vi "GetControlSpecificLocalizedPhrase.vi"(7 "Dictionary":T2, 8 "error in (no error)":errorcluster, 9 "Font Info":T1, 10 "Target Language":string, 11 "Control Reference":refnum<vi>) -> (0 "error out":errorcluster, 3 "Control ref out":refnum<vi>)   [LabVIEW 2019]
uses:
  Dictionary--Cluster.ctl
  Font -- Cluster.ctl
  Phrase Dictionary Entry -- Cluster.ctl
  Font Info -- Cluster.ctl
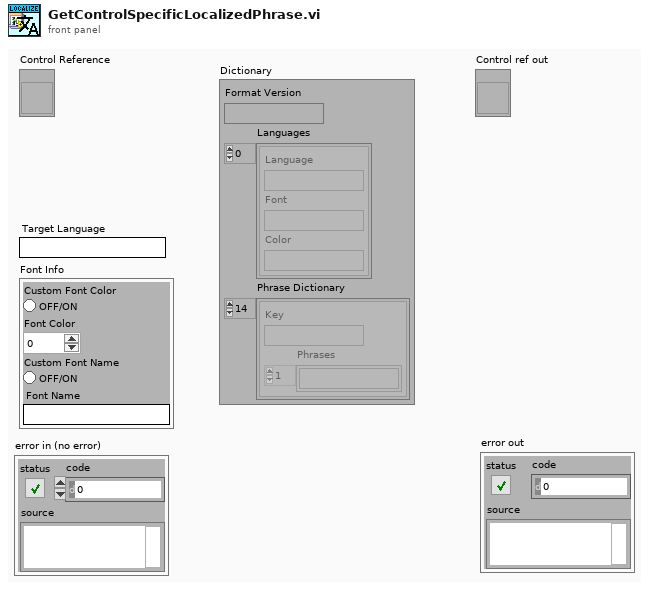
[diagram p1: front panel]
types:
  T1 = typedef "Font Info -- Cluster.ctl" = cluster{"Custom Font Color":bool, "Font Color":u32, "Custom Font Name":bool, "Font Name":string}
  T2 = typedef "Dictionary--Cluster.ctl" = cluster{"Format Version":string, "Languages":T3[], "Phrase Dictionary":T4[]}
  T3 = typedef "Font -- Cluster.ctl" = cluster{"Language":string, "Font":string, "Color":string}
  T4 = typedef "Phrase Dictionary Entry -- Cluster.ctl" = cluster{"Key":string, "Phrases":string[]}
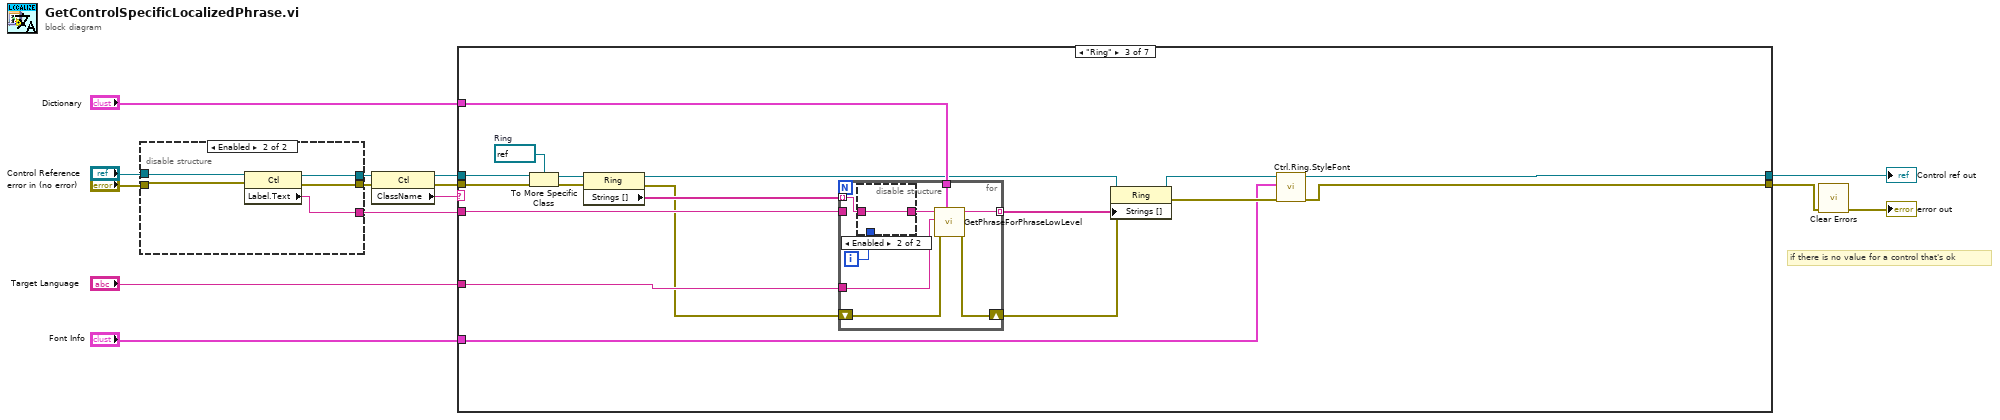
[diagram p0: block diagram]
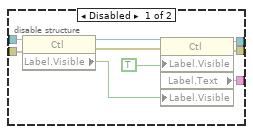
[diagram p2: hidden frame]
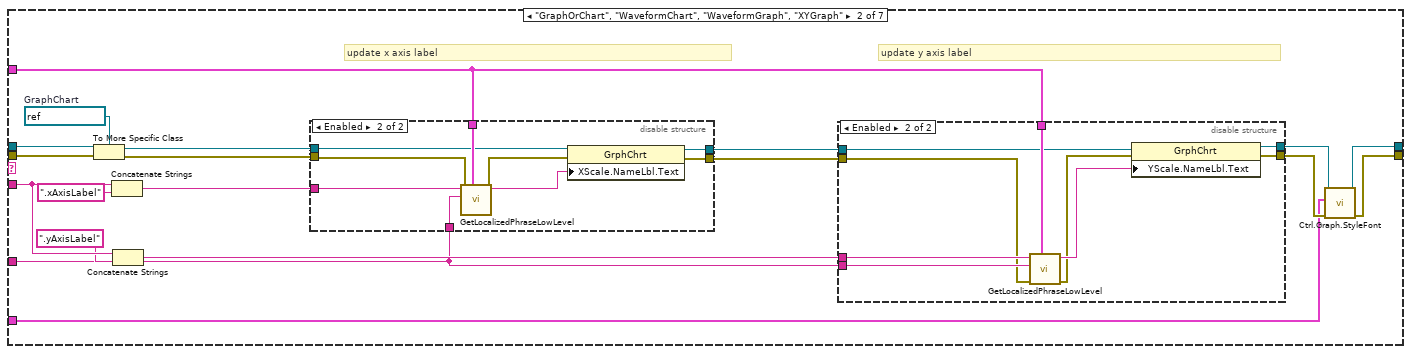
[diagram p4: hidden frame]
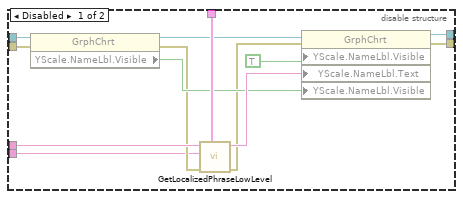
[diagram p5: hidden frame]
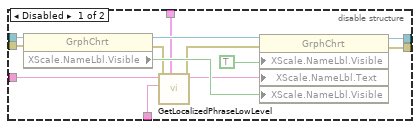
[diagram p6: hidden frame]
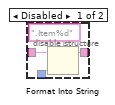
[diagram p7: hidden frame]
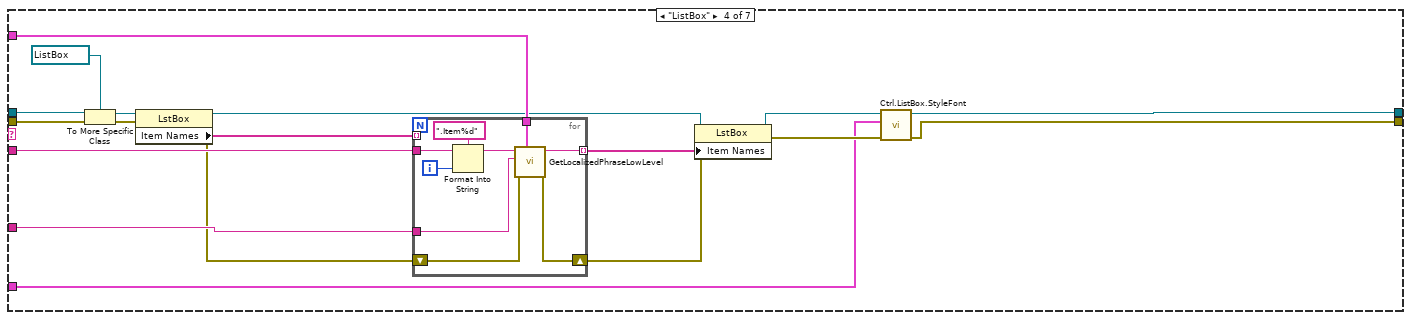
[diagram p8: hidden frame]
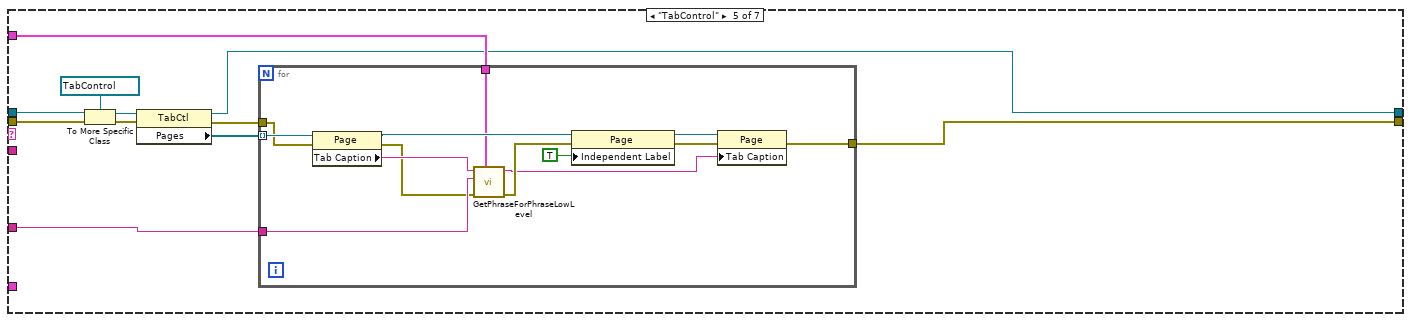
[diagram p9: hidden frame]
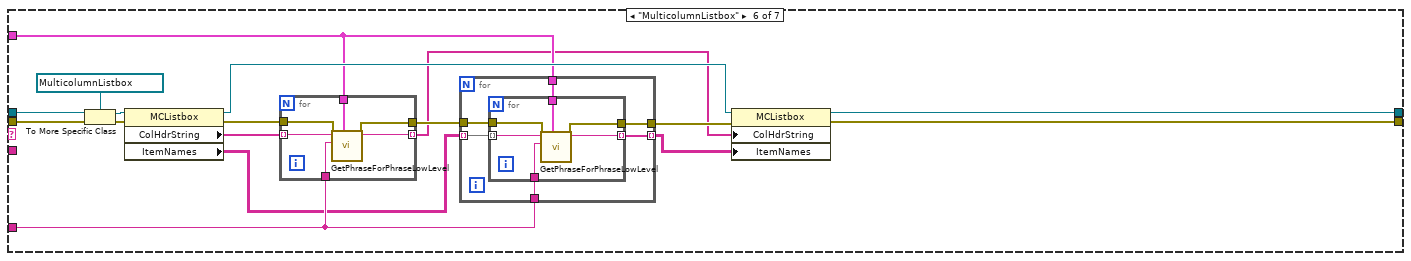
[diagram p10: hidden frame]
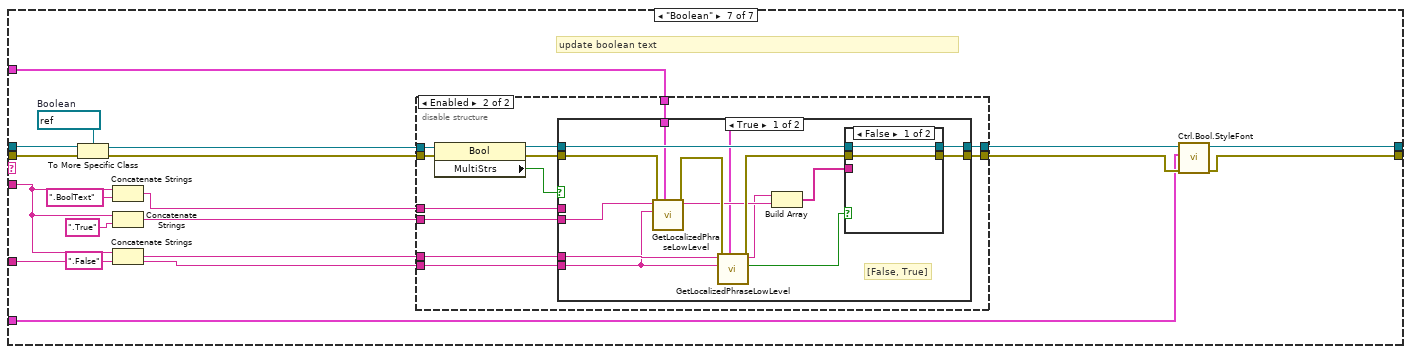
[diagram p11: hidden frame]
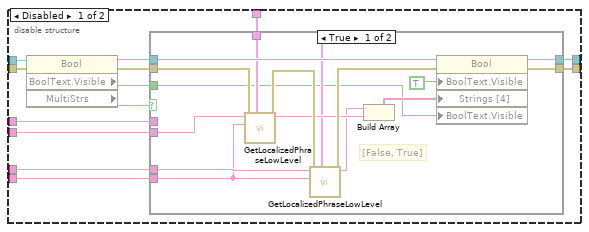
[diagram p12: hidden frame]
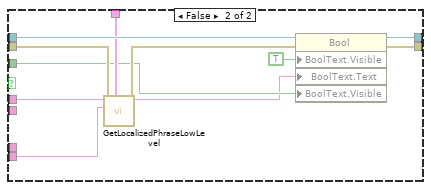
[diagram p13: hidden frame]
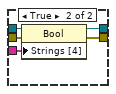
[diagram p14: hidden frame]
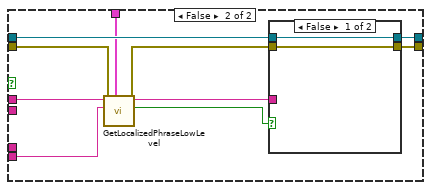
[diagram p15: hidden frame]
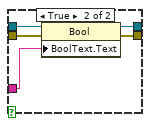
[diagram p16: hidden frame]
diagram:
  # "if there is no value for a control that's ok"
  n1 = disable-structure shown="Enabled" {
    disable-tunnel: "Control Reference" -> [w19 w24]
    disable-tunnel: [w18 w28] -> w12
    disable-tunnel: [w17 w27] -> w11
    disable-tunnel: [w16 w26] -> w8
    disable-tunnel: "error in (no error)" -> [w15 w25]
    frame Disabled {
      n2 = property on="Property Node" class="Ctl"(reference=w19, error in=w15) -> (reference out=w23:refnum<vi>, error out=w20:errorcluster, "Label.Visible"=w22:bool)
      n3 = property on="Property Node" class="Ctl"(reference=w23, error in=w20, "Label.Visible"=TRUE, "Label.Visible"=w22) -> (reference out=w18:refnum<vi>, error out=w16:errorcluster, "Label.Text"=w17:string)
    }
    frame Enabled {
      n4 = property on="Property Node" class="Ctl"(reference=w24, error in=w25) -> (reference out=w28:refnum<vi>, error out=w26:errorcluster, "Label.Text"=w27:string)
    }
  }
  n5 = property on="Property Node" class="Ctl"(reference=w12, error in=w8) -> (reference out=w10:refnum<vi>, error out=w7:errorcluster, "ClassName"=w14:string)
  n6 = case shown="\"Ring\"" w14 {
    tunnel: w11 -> [_ w44 w105 w137 _ _ w213]
    tunnel: w10 -> [w30 w48 w110 w142 w162 w192 w229]
    tunnel: "Dictionary" -> [_ w41 w104 w136 w155 w180 w222]
    tunnel: "Target Language" -> [_ w38 w103 w135 w156 w179 w221]
    tunnel: w7 -> [w29 w40 w109 w141 w161 w191 w224]
    tunnel: [w30 w35 w97 w127 w154 w185 w219] -> w6
    tunnel: [w29 w33 w95 w128 w152 w183 w217] -> w3
    tunnel: "Font Info" -> [_ w32 w94 w125 _ _ w216]
    frame "0", Default {
    }
    frame "GraphOrChart", "WaveformChart", "WaveformGraph", "XYGraph" {
      w46 = refnum<vi> refnum  # GraphChart
      # "update y axis label"
      # "update x axis label"
      n7 = To More Specific Class(target class=w46, reference=w48, error in=w40) -> (specific class reference=w47:refnum<vi>, error out=w39:errorcluster)
      n8 = Concatenate Strings(w44, ".xAxisLabel" ("string")) -> (w45:string)
      n9 = Concatenate Strings(w44, ".yAxisLabel" ("string")) -> (w42:string)
      n10 = disable-structure shown="Enabled" {
        disable-tunnel: w47 -> [w84 w85]
        disable-tunnel: w45 -> [w82 w93]
        disable-tunnel: w41 -> [w78 w91]
        disable-tunnel: w39 -> [w77 w86]
        disable-tunnel: w38 -> [w74 w89]
        disable-tunnel: [w73 w88] -> w37
        disable-tunnel: [w72 w87] -> w31
        frame Disabled {
          n11 = property class="GrphChrt"(reference=w84, error in=w77) -> (reference out=w79:refnum<vi>, error out=w76:errorcluster, "XScale.NameLbl.Visible"=w83:bool)
          n12 = call "GetLocalizedPhraseLowLevel.vi"("Dictionary"=w78, "error in (no error)"=w76, "Target Language"=w74, "Key"=w82) -> ("error out"=w75:errorcluster, "Localized Phrase"=w81:string)  [unwired: 5 in, 1 out]
          n13 = property class="GrphChrt"(reference=w79, error in=w75, "XScale.NameLbl.Visible"=TRUE ("X Scale.Name Label.Visible"), "XScale.NameLbl.Text"=w81, "XScale.NameLbl.Visible"=w83) -> (reference out=w73:refnum<vi>, error out=w72:errorcluster)
        }
        frame Enabled {
          n14 = call "GetLocalizedPhraseLowLevel.vi"("Dictionary"=w91, "error in (no error)"=w86, "Target Language"=w89, "Key"=w93) -> ("error out"=w90:errorcluster, "Localized Phrase"=w92:string)  [unwired: 5 in, 1 out]
          n15 = property class="GrphChrt"(reference=w85, error in=w90, "XScale.NameLbl.Text"=w92) -> (reference out=w88:refnum<vi>, error out=w87:errorcluster)
        }
      }
      n16 = disable-structure shown="Enabled" {
        disable-tunnel: w42 -> [w62 w71]
        disable-tunnel: w41 -> [w61 w70]
        disable-tunnel: w38 -> [w54 w67]
        disable-tunnel: w37 -> [w53 w63]
        disable-tunnel: [w52 w66] -> w36
        disable-tunnel: [w51 w65] -> w34
        disable-tunnel: w31 -> [w50 w64]
        frame Disabled {
          n17 = property class="GrphChrt"(reference=w53, error in=w50) -> (reference out=w60:refnum<vi>, error out=w56:errorcluster, "YScale.NameLbl.Visible"=w57:bool)
          n18 = call "GetLocalizedPhraseLowLevel.vi"("Dictionary"=w61, "error in (no error)"=w56, "Target Language"=w54, "Key"=w62) -> ("error out"=w55:errorcluster, "Localized Phrase"=w58:string)  [unwired: 5 in, 1 out]
          n19 = property class="GrphChrt"(reference=w60, error in=w55, "YScale.NameLbl.Visible"=TRUE ("X Scale.Name Label.Visible"), "YScale.NameLbl.Text"=w58, "YScale.NameLbl.Visible"=w57) -> (reference out=w52:refnum<vi>, error out=w51:errorcluster)
        }
        frame Enabled {
          n20 = call "GetLocalizedPhraseLowLevel.vi"("Dictionary"=w70, "error in (no error)"=w64, "Target Language"=w67, "Key"=w71) -> ("error out"=w68:errorcluster, "Localized Phrase"=w69:string)  [unwired: 5 in, 1 out]
          n21 = property class="GrphChrt"(reference=w63, error in=w68, "YScale.NameLbl.Text"=w69) -> (reference out=w66:refnum<vi>, error out=w65:errorcluster)
        }
      }
      n22 = call "Ctrl.Graph.StyleFont.vi"("error in (no error)"=w34, "Font Info"=w32, "Graph Ctrl Ref in"=w36) -> ("error out"=w33:errorcluster, "Graph Ctrl Ref out"=w35:refnum<vi>)  [unwired: 7 in]
    }
    frame "Ring" {
      w111 = refnum<vi> refnum  # Ring
      n23 = To More Specific Class(target class=w111, reference=w110, error in=w109) -> (specific class reference=w108:refnum<vi>, error out=w107:errorcluster)
      n24 = property class="Ring"(reference=w108, error in=w107) -> (reference out=w101:refnum<vi>, error out=w100:errorcluster, "Strings []"=w106:string[])
      n25 = for {
        tunnel: w106 -> [w112] mode=indexing
        tunnel: w105 -> [_]
        tunnel: w104 -> [w118]
        shift-right: [w117] -> w99
        shift-left: w100 -> [w114]
        tunnel: w103 -> [w113]
        tunnel: [w115] -> w102 mode=indexing
        i -> [w119]
        n26 = disable-structure shown="Enabled" {
          disable-tunnel: w112 -> [w123 w124]
          disable-tunnel: w119 -> [w121 _]
          disable-tunnel: [w120 w124] -> w116
          frame Disabled {
            n27 = Format Into String(format string=".Item%d", initial string=w123, w121) -> (resulting string=w120:string)  [unwired: 1 in, 1 out]
          }
          frame Enabled {
          }
        }
        n28 = call "GetPhraseForPhraseLowLevel.vi"("Dictionary"=w118, "error in (no error)"=w114, "Target Language"=w113, "Phrase"=w116) -> ("error out"=w117:errorcluster, "Phrase In Target Language"=w115:string)  [unwired: 6 in]
      }
      n29 = property class="Ring"(reference=w101, error in=w99, "Strings []"=w102) -> (reference out=w98:refnum<vi>, error out=w96:errorcluster)
      n30 = call "Ctrl.Ring.StyleFont.vi"("error in (no error)"=w96, "Font Info"=w94, "Ring Ref in"=w98) -> ("error out"=w95:errorcluster, "Ring Ref out"=w97:refnum<vi>)  [unwired: 7 in]
    }
    frame "ListBox" {
      n31 = To More Specific Class(target class=refnum<vi> refnum ("reference out"), reference=w142, error in=w141) -> (specific class reference=w140:refnum<vi>, error out=w139:errorcluster)
      n32 = property class="LstBox"(reference=w140, error in=w139) -> (reference out=w133:refnum<vi>, error out=w132:errorcluster, "Item Names"=w138:string[])
      n33 = for {
        tunnel: w138 -> [_] mode=indexing
        tunnel: w137 -> [w151]
        tunnel: w136 -> [w148]
        shift-right: [w147] -> w131
        shift-left: w132 -> [w144]
        tunnel: w135 -> [w143]
        tunnel: [w145] -> w134 mode=indexing
        i -> [w149]
        n34 = Format Into String(format string=".Item%d", initial string=w151, w149) -> (resulting string=w146:string)  [unwired: 1 in, 1 out]
        n35 = call "GetLocalizedPhraseLowLevel.vi"("Dictionary"=w148, "error in (no error)"=w144, "Target Language"=w143, "Key"=w146) -> ("error out"=w147:errorcluster, "Localized Phrase"=w145:string)  [unwired: 5 in, 1 out]
      }
      n36 = property class="LstBox"(reference=w133, error in=w131, "Item Names"=w134) -> (reference out=w126:refnum<vi>, error out=w129:errorcluster)
      n37 = call "Ctrl.ListBox.StyleFont.vi"("error in (no error)"=w129, "Font Info"=w125, "Listbox Ref"=w126) -> ("error out"=w128:errorcluster, "Listbox Ref out"=w127:refnum<vi>)  [unwired: 7 in]
    }
    frame "TabControl" {
      n38 = To More Specific Class(target class=refnum<vi> refnum ("reference out"), reference=w162, error in=w161) -> (specific class reference=w160:refnum<vi>, error out=w159:errorcluster)
      n39 = property class="TabCtl"(reference=w160, error in=w159) -> (reference out=w154:refnum<vi>, error out=w153:errorcluster, "Pages"=w157:refnum<vi>[])
      n40 = for {
        tunnel: w157 -> [w173] mode=indexing
        tunnel: w156 -> [w168]
        tunnel: w155 -> [w170]
        tunnel: w153 -> [w171]
        tunnel: [w164] -> w152
        n41 = property class="Page"(reference=w173, error in=w171) -> (reference out=w172:refnum<vi>, error out=w167:errorcluster, "Tab Caption"=w169:string)
        n42 = call "GetPhraseForPhraseLowLevel.vi"("Dictionary"=w170, "error in (no error)"=w167, "Target Language"=w168, "Phrase"=w169) -> ("error out"=w166:errorcluster, "Phrase In Target Language"=w163:string)  [unwired: 6 in]
        n43 = property class="Page"(reference=w172, error in=w166, "Independent Label"=TRUE) -> (reference out=w175:refnum<vi>, error out=w165:errorcluster)
        n44 = property class="Page"(reference=w175, error in=w165, "Tab Caption"=w163) -> (error out=w164:errorcluster)  [unwired: 1 out]
      }
    }
    frame "MulticolumnListbox" {
      n45 = To More Specific Class(target class=refnum<vi> refnum ("reference out"), reference=w192, error in=w191) -> (specific class reference=w190:refnum<vi>, error out=w189:errorcluster)
      n46 = property class="MCListbox"(reference=w190, error in=w189) -> (reference out=w186:refnum<vi>, error out=w184:errorcluster, "ColHdrString"=w187:string[], "ItemNames"=w177:string[][])
      n47 = for {
        tunnel: w187 -> [w210] mode=indexing
        tunnel: w179 -> [w209]
        tunnel: w180 -> [w208]
        tunnel: [w207] -> w178 mode=indexing
        tunnel: w184 -> [w206]
        tunnel: [w205] -> w182
        n48 = call "GetPhraseForPhraseLowLevel.vi"("Dictionary"=w208, "error in (no error)"=w206, "Target Language"=w209, "Phrase"=w210) -> ("error out"=w205:errorcluster, "Phrase In Target Language"=w207:string)  [unwired: 6 in]
      }
      n49 = for {
        tunnel: w182 -> [w198]
        tunnel: [w197] -> w181
        tunnel: w180 -> [w196]
        tunnel: w179 -> [w195]
        tunnel: w177 -> [w194] mode=indexing
        tunnel: [w193] -> w176 mode=indexing
        n50 = for {
          tunnel: w194 -> [w204] mode=indexing
          tunnel: w195 -> [w203]
          tunnel: w196 -> [w202]
          tunnel: [w201] -> w193 mode=indexing
          tunnel: w198 -> [w200]
          tunnel: [w199] -> w197
          n51 = call "GetPhraseForPhraseLowLevel.vi"("Dictionary"=w202, "error in (no error)"=w200, "Target Language"=w203, "Phrase"=w204) -> ("error out"=w199:errorcluster, "Phrase In Target Language"=w201:string)  [unwired: 6 in]
        }
      }
      n52 = property class="MCListbox"(reference=w186, error in=w181, "ColHdrString"=w178, "ItemNames"=w176) -> (reference out=w185:refnum<vi>, error out=w183:errorcluster)
    }
    frame "Boolean" {
      w227 = refnum<vi> refnum  # Boolean
      # "update boolean text"
      n53 = To More Specific Class(target class=w227, reference=w229, error in=w224) -> (specific class reference=w228:refnum<vi>, error out=w223:errorcluster)
      n54 = Concatenate Strings(w213, ".BoolText" ("string")) -> (w211:string)
      n55 = Concatenate Strings(w213, ".True" ("string")) -> (w226:string)
      n56 = Concatenate Strings(w213, ".False" ("string")) -> (w225:string)
      n57 = disable-structure shown="Enabled" {
        disable-tunnel: w228 -> [w242 w280]
        disable-tunnel: w226 -> [w241 w279]
        disable-tunnel: w225 -> [w239 w277]
        disable-tunnel: w223 -> [w238 w276]
        disable-tunnel: w222 -> [w236 w274]
        disable-tunnel: w221 -> [w233 w272]
        disable-tunnel: [w232 w271] -> w220
        disable-tunnel: [w231 w270] -> w218
        disable-tunnel: w211 -> [w230 w269]
        frame Disabled {
          n58 = property class="Bool"(reference=w242, error in=w238) -> (reference out=w240:refnum<vi>, error out=w237:errorcluster, "BoolText.Visible"=w235:bool, "MultiStrs"=w234:bool)
          n59 = case shown="True" w234 {
            tunnel: w241 -> [w257 _]
            tunnel: w240 -> [w256 w268]
            tunnel: w239 -> [w255 _]
            tunnel: w233 -> [w244 w258]
            tunnel: w237 -> [w254 w267]
            tunnel: w236 -> [w250 w265]
            tunnel: w235 -> [w247 w263]
            tunnel: w230 -> [_ w262]
            tunnel: [w246 w260] -> w232
            tunnel: [w245 w259] -> w231
            frame True {
              # "[False, True]"
              n60 = call "GetLocalizedPhraseLowLevel.vi"("Dictionary"=w250, "error in (no error)"=w254, "Target Language"=w244, "Key"=w257) -> ("error out"=w253:errorcluster, "Localized Phrase"=w251:string)  [unwired: 5 in, 1 out]
              n61 = call "GetLocalizedPhraseLowLevel.vi"("Dictionary"=w250, "error in (no error)"=w253, "Target Language"=w244, "Key"=w255) -> ("error out"=w252:errorcluster, "Localized Phrase"=w243:string)  [unwired: 5 in, 1 out]
              n62 = Build Array(w243, w251) -> (w249:string[])
              n63 = property class="Bool"(reference=w256, error in=w252, "BoolText.Visible"=TRUE ("X Scale.Name Label.Visible"), "Strings [4]"=w249, "BoolText.Visible"=w247) -> (reference out=w246:refnum<vi>, error out=w245:errorcluster)
            }
            frame False {
              n64 = call "GetLocalizedPhraseLowLevel.vi"("Dictionary"=w265, "error in (no error)"=w267, "Target Language"=w258, "Key"=w262) -> ("error out"=w266:errorcluster, "Localized Phrase"=w261:string)  [unwired: 5 in, 1 out]
              n65 = property class="Bool"(reference=w268, error in=w266, "BoolText.Visible"=TRUE ("X Scale.Name Label.Visible"), "BoolText.Text"=w261, "BoolText.Visible"=w263) -> (reference out=w260:refnum<vi>, error out=w259:errorcluster)
            }
          }
        }
        frame Enabled {
          n66 = property class="Bool"(reference=w280, error in=w276) -> (reference out=w278:refnum<vi>, error out=w275:errorcluster, "MultiStrs"=w273:bool)
          n67 = case shown="True" w273 {
            tunnel: w279 -> [w294 _]
            tunnel: w278 -> [w293 w311]
            tunnel: w277 -> [w292 _]
            tunnel: w272 -> [w283 w303]
            tunnel: w275 -> [w291 w310]
            tunnel: w274 -> [w287 w308]
            tunnel: w269 -> [_ w307]
            tunnel: [w285 w305] -> w271
            tunnel: [w284 w304] -> w270
            frame True {
              # "[False, True]"
              n68 = call "GetLocalizedPhraseLowLevel.vi"("Dictionary"=w287, "error in (no error)"=w291, "Target Language"=w283, "Key"=w294) -> ("error out"=w290:errorcluster, "Localized Phrase"=w288:string)  [unwired: 5 in, 1 out]
              n69 = call "GetLocalizedPhraseLowLevel.vi"("Dictionary"=w287, "error in (no error)"=w290, "Target Language"=w283, "Key"=w292) -> ("error out"=w289:errorcluster, "Key Present?"=w281:bool, "Localized Phrase"=w282:string)  [unwired: 5 in]
              n70 = Build Array(w282, w288) -> (w286:string[])
              n71 = case shown="False" w281 {
                tunnel: w293 -> [w296 w301]
                tunnel: w289 -> [w295 w300]
                tunnel: w286 -> [_ w299]
                tunnel: [w296 w298] -> w285
                tunnel: [w295 w297] -> w284
                frame False {
                }
                frame True {
                  n72 = property class="Bool"(reference=w301, error in=w300, "Strings [4]"=w299) -> (reference out=w298:refnum<vi>, error out=w297:errorcluster)
                }
              }
            }
            frame False {
              n73 = call "GetLocalizedPhraseLowLevel.vi"("Dictionary"=w308, "error in (no error)"=w310, "Target Language"=w303, "Key"=w307) -> ("error out"=w309:errorcluster, "Key Present?"=w302:bool, "Localized Phrase"=w306:string)  [unwired: 5 in]
              n74 = case shown="False" w302 {
                tunnel: w311 -> [w313 w318]
                tunnel: w309 -> [w312 w317]
                tunnel: w306 -> [_ w316]
                tunnel: [w313 w315] -> w305
                tunnel: [w312 w314] -> w304
                frame False {
                }
                frame True {
                  n75 = property class="Bool"(reference=w318, error in=w317, "BoolText.Text"=w316) -> (reference out=w315:refnum<vi>, error out=w314:errorcluster)
                }
              }
            }
          }
        }
      }
      n76 = call "Ctrl.Bool.StyleFont.vi"("error in (no error)"=w218, "Font Info"=w216, "Bool Ref in"=w220) -> ("error out"=w217:errorcluster, "Bool Ref out"=w219:refnum<vi>)  [unwired: 7 in]
    }
  }
  "Control ref out" <- w6
  n77 = call <vilib>:"Clear Errors.vi"("error in (no error)"=w3) -> ("error out"=→"error out":errorcluster)  [unwired: 5 in, 1 out]
